vi "TestHelioscanRoutine.vi"() -> ()   [LabVIEW 2010]
uses:
  <vilib>/Instr/_visa.llb/VISA Configure Serial Port (Instr).vi
panel:
  out "concatenated string 2":string
  out "read buffer":string
  out "Serial Settings:Number of Bytes at Serial Port":u32
  in  "error in (no error) 2":errorcluster
  out "concatenated string":string
  out "approved response?":bool
  out "read string":string
  in  "string to write":string
  out "error out":errorcluster
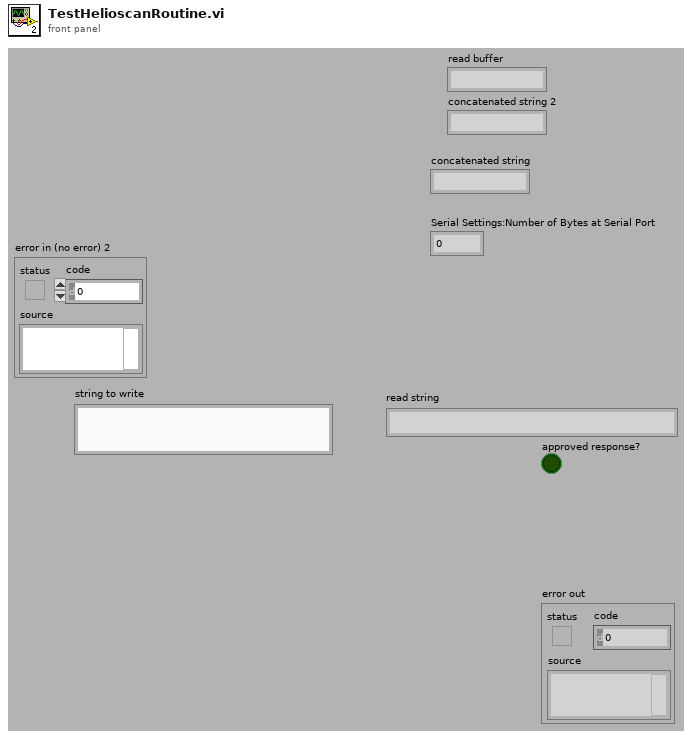
[diagram p1: front panel]
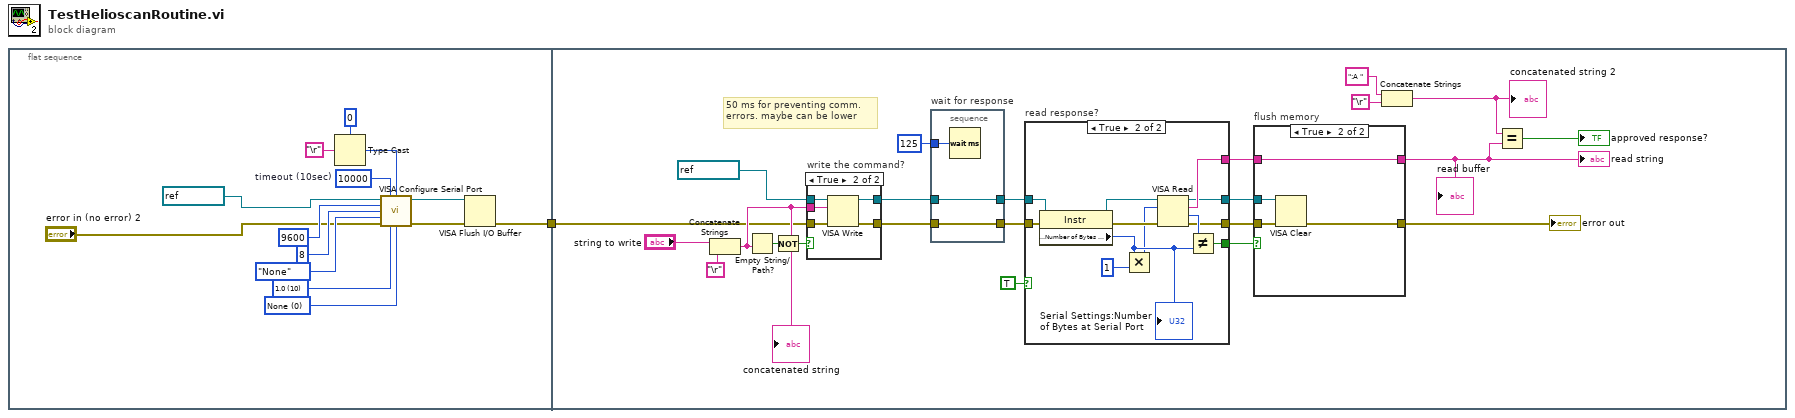
[diagram p0: block diagram]
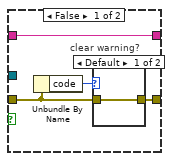
[diagram p2: hidden frame]
diagram:
  n1 = flat-sequence {
    tunnel: [w2] -> w1
    tunnel: w1 -> [w18]
    frame #0 {
      w10 = u16 0 items=["None", "XON/XOFF", "RTS/CTS", "XON/XOFF & RTS/CTS", "DTR/DSR", "XON/XOFF & DTR/DSR"] ("flow control (0:none)")
      w11 = u16 10 items=["1.0"=10, "1.5"=15, "2.0"=20] ("stop bits (10: 1 bit)")
      w15 = u32 10000  # timeout (10sec)
      n2 = Type Cast(type=u8 0, x="\r") -> (*(type *) &x=w6:u8)
      n3 = call-poly "VISA Configure Serial Port"("VISA resource name"=refnum<visa-resource-name> "COM3", "timeout (10sec)"=w15, "termination char\n(0xA = '\\n' = LF)"=w6, "baud rate (9600)"=u32 9600, "data bits (8)"=u16 8, "parity (0:none)"=enum16{"None", "Odd", "Even", "Mark", "Space"}."None", "error in (no error)"="error in (no error) 2", "stop bits (10: 1 bit)"=w11, "flow control (0:none)"=w10) -> ("VISA resource name out"=w9:refnum<visa-resource-name>, "error out"=w8:errorcluster)  [unwired: 5 in]
      n4 = VISA Flush I/O Buffer(VISA resource name=w9, error in (no error)=w8) -> (error out=w2:errorcluster)  [unwired: 1 in, 1 out]
    }
    frame #1 {
      # "50 ms for preventing comm.\nerrors. maybe can be lower"
      n5 = Concatenate Strings("string to write", "\r") -> (w31:string)
      "concatenated string" <- w31
      n6 = Empty String/Path?(string/path=w31) -> (empty?=w33:bool)
      n7 = Not(x=w33) -> (.not. x?=w32:bool)
      n8 = case "write the command?" shown="True" w32 {
        tunnel: [w66 w71] -> w29
        tunnel: refnum<visa-resource-name> "COM3" ("VISA resource name") -> [w65 w70]
        tunnel: w18 -> [w66 w69]
        tunnel: [w65 w68] -> w30
        tunnel: w31 -> [_ w67]
        frame False {
        }
        frame True {
          n9 = VISA Write(VISA resource name=w70, write buffer=w67, error in (no error)=w69) -> (VISA resource name out=w68:refnum<visa-resource-name>, error out=w71:errorcluster)  [unwired: 1 out]
        }
      }
      n10 = stacked-sequence "wait for response" {
        tunnel: w29 -> [w64]
        tunnel: [w64] -> w26
        tunnel: w30 -> [w63]
        tunnel: [w63] -> w27
        tunnel: u32 125 ("delay before read (ms)") -> [w62]
        frame #0 {
          n11 = Wait (ms)(milliseconds to wait=w62) -> ()  [unwired: 1 out]
        }
      }
      n12 = case "read response?" shown="True" TRUE {
        tunnel: w26 -> [w49 w59]
        tunnel: [w49 w53] -> w23
        tunnel: w27 -> [w48 w61]
        tunnel: [_ w57] -> w24
        tunnel: [_ w55] -> w22
        tunnel: [w48 w54] -> w25
        frame False {
        }
        frame True {
          n13 = property class="Instr"(reference=w61, error in=w59) -> (reference out=w60:refnum<visa-resource-name>, error out=w58:errorcluster, "Serial Settings:Number of Bytes at Serial Port"=w52:u32)
          "Serial Settings:Number of Bytes at Serial Port" <- w52
          n14 = Multiply(x=w52, y=u32 1) -> (x*y=w50:u32)
          n15 = VISA Read(VISA resource name=w60, byte count=w50, error in (no error)=w58) -> (VISA resource name out=w54:refnum<visa-resource-name>, read buffer=w57:string, return count=w56:u32, error out=w53:errorcluster)
          n16 = Not Equal?(x=w56, y=w52) -> (x != y?=w55:bool)
        }
      }
      n17 = case "flush memory" shown="True" w22 {
        tunnel: w23 -> [w40 w47]
        tunnel: w25 -> [_ w46]
        tunnel: [w42 w45] -> w36
        tunnel: w24 -> [w42 w45]
        tunnel: [w39 w44] -> w38
        frame False {
          n18 = Unbundle By Name(w40) -> ("code"=w41:i32)
          n19 = case "clear warning?" shown="Default" w41 {
            tunnel: w40 -> [w43 _]
            tunnel: [w43 _] -> w39
            frame Default {
            }
            frame 1073676294 {
            }
          }
        }
        frame True {
          n20 = VISA Clear(VISA resource name=w46, error in (no error)=w47) -> (error out=w44:errorcluster)  [unwired: 1 out]
        }
      }
      "error out" <- w38
      "read string" <- w36
      "read buffer" <- w36
      n21 = Concatenate Strings "Concatenate Strings"(":A " ("y"), "\r") -> (w16:string)
      "concatenated string 2" <- w16
      n22 = Equal?(x=w16, y=w36) -> (x = y?=→"approved response?":bool)
    }
  }
